vi "Hello World.vi"   [LabVIEW 2018]
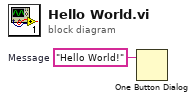
[diagram p0: block diagram]
diagram:
  w1 = "Hello World!"  # Message
  n1 = One Button Dialog(message=w1) -> ()  [unwired: 1 in, 1 out]
